vi "Write To Spreadsheet File2.vi"(0 "delimiter (\\t)":string="\t", 1 "transpose? (no:F)":bool, 4 "format (%d)":string="%d", 5 "append to file? (new file:F)":bool, 6 "1D data":i64[](array[numeric]), 7 "2D data":ext[][](array[numeric]), 8 "file path (dialog if empty)":path) -> (3 "new file path (Not A Path if cancelled)":path)   [LabVIEW 2015]
doc: "Converts a 2D or 1D array of strings, signed integers, or double-precision numbers to a text string and writes the string to a new byte stream file or appends the string to an existing file. Wire data to the <B>2D data</B> input or <B>1D data</B> input to determine the polymorphic instance to use or manually select the instance.\n\nUse this VI to transpose or separate data.\n\n<B>Note</B> To format with Microsoft Excel, use ActiveX with LabVIEW or the Report Generation Toolkit for Microsoft Office."
uses:
  <vilib>/Utility/error.llb/DialogType.ctl
panel:
  in  "prompt":string="Choose file to write."
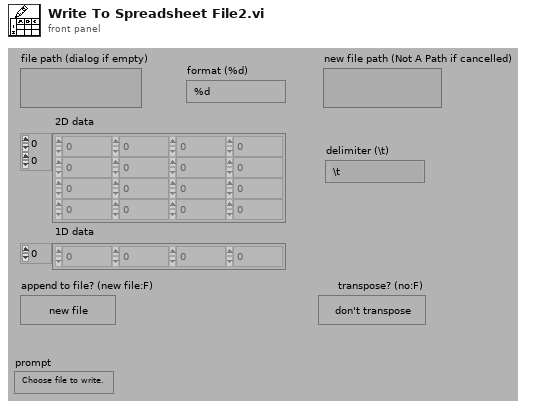
[diagram p1: front panel]
types:
  T1 = typedef "DialogType.ctl" = u16
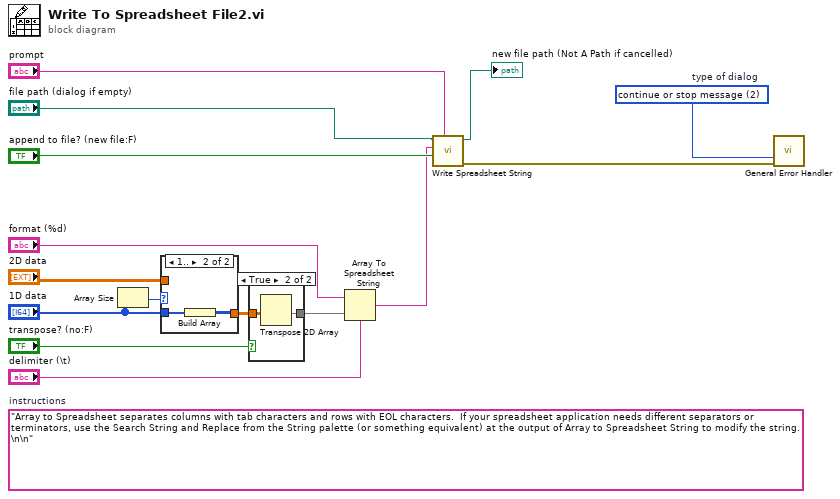
[diagram p0: block diagram]
diagram:
  w2 = T1 2 items=["no dialog", "OK message", "continue or stop message", "OK message + warnings", "continue/stop + warnings"]  # type of dialog
  (unwired) "Array to Spreadsheet separates columns with tab characters and rows with EOL characters.  If your spreadsheet application needs different separators or terminators, use the Search String and Replace from the String palette (or something equivalent) at the output of Array to Spreadsheet String to modify the string.\n\n"  # instructions
  n1 = Array Size(array="1D data") -> (size(s)=w15:i32)
  n2 = case shown="1.." w15 {
    tunnel: "1D data" -> [_ w18]
    tunnel: [w16 w17] -> w11
    tunnel: "2D data" -> [w16 _]
    frame ..0 {
      # "1D array is empty"
    }
    frame 1.. {
      n3 = Build Array(w18) -> (w17:i64[][])
    }
  }
  n4 = case shown="True" "transpose? (no:F)" {
    tunnel: [w19 w21] -> w9
    tunnel: w11 -> [w19 w20]
    frame False {
    }
    frame True {
      n5 = Transpose 2D Array(2D array=w20) -> (transposed array=w21:ext[][])
    }
  }
  n6 = Array To Spreadsheet String(delimiter (Tab)="delimiter (\\t)", array=w9, 3:"format (%d)") -> (spreadsheet string=w4:string)
  n7 = call <vilib>:"Write Spreadsheet String.vi"("prompt"="prompt", "append to file? (new file:F)"="append to file? (new file:F)", "spreadsheet string"=w4, "file path (dialog if empty)"="file path (dialog if empty)") -> ("error out"=w1:errorcluster, "path"=→"new file path (Not A Path if cancelled)":path)  [unwired: 6 in]
  n8 = call <vilib>:"General Error Handler.vi"("type of dialog (OK msg:1)"=w2, "error in (no error)"=w1) -> ()  [unwired: 9 in, 5 out]
